vi "Open Listener.vi"(8 "error in (no error)":errorcluster, 11 "Messaging Server Module in":refnum<class "Messaging Server Module.lvclass">) -> (0 "error out":errorcluster, 3 "Messaging Server Module out":refnum<class "Messaging Server Module.lvclass">)   [LabVIEW 2020, in "Volatus.lvlib" / "Messaging Server Module.lvclass"]
uses:
  Messaging Server Module.lvclass
  Messaging Server Module.lvclass/Messaging Server Module.ctl
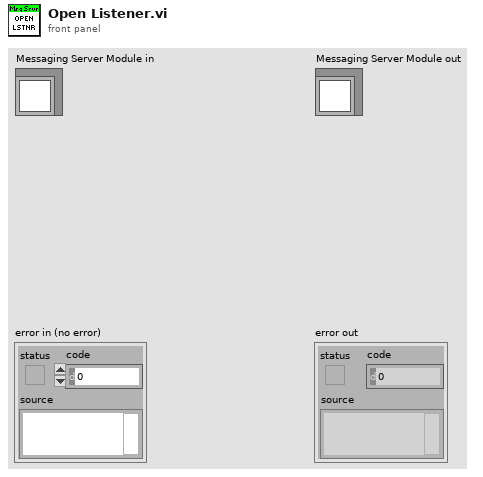
[diagram p1: front panel]
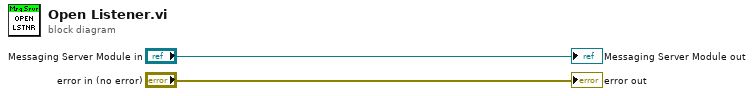
[diagram p0: block diagram]
diagram:
  "error out" <- "error in (no error)"
  "Messaging Server Module out" <- "Messaging Server Module in"
